vi "solar_visa VISA Open.vi"(6 "Access Mode (0)":T1 items=["VISA Defaults"=0, "Exclusive Lock"=1, "Load Configured Settings"=4], 8 "error in (no error)":errorcluster, 9 "VISA Close? (T)":bool=TRUE, 10 "VISA Timeout (0 = Ignore)":u32, 11 "VISA Resource in":refnum<visa-resource-name>) -> (0 "error out":errorcluster, 3 "VISA Resource out":refnum<visa-resource-name>)   [LabVIEW 2018]
doc: "This opens a VISA session. \nIf <b>VISA Close?</b> is true the previous VISA session is closed. \nIf <b>VISA Timeout</b> is greater than 0 the VISA timeout is set."
uses:
  <vilib>/Instr/_visa.llb/VISA Open Access Mode.ctl
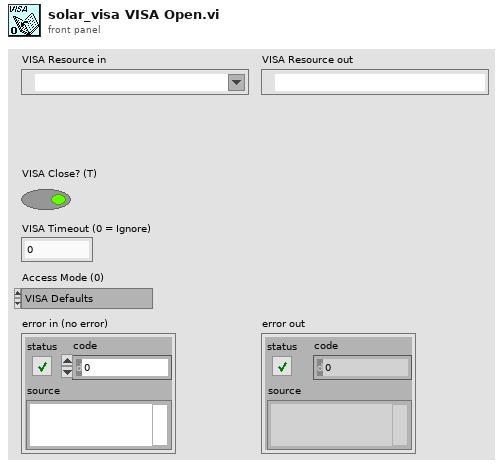
[diagram p1: front panel]
types:
  T1 = typedef "VISA Open Access Mode.ctl" = u32
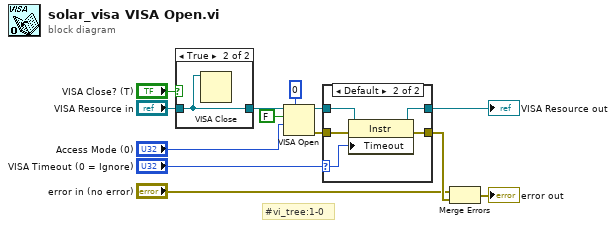
[diagram p0: block diagram]
diagram:
  # "#vi_tree:1-0"
  n1 = case shown="True" "VISA Close? (T)" {
    tunnel: "VISA Resource in" -> [w14 w15]
    tunnel: [w14 w15] -> w2
    frame False {
    }
    frame True {
      n2 = VISA Close(VISA resource name=w15) -> ()  [unwired: 1 in, 1 out]
    }
  }
  n3 = VISA Open(timeout (0)=u32 0 ("VISA Open timeout (0)"), duplicate session (F)=FALSE, access mode="Access Mode (0)", VISA resource name=w2) -> (VISA resource name=w1:refnum<visa-resource-name>, error out=w5:errorcluster)  [unwired: 1 in]
  n4 = case shown="Default" "VISA Timeout (0 = Ignore)" {
    selector: "VISA Timeout (0 = Ignore)" -> [_ w18]
    tunnel: w5 -> [w16 w22]
    tunnel: [w16 w21] -> w10
    tunnel: w1 -> [w17 w20]
    tunnel: [w17 w19] -> w9
    frame 0 {
    }
    frame Default {
      n5 = property class="Instr"(reference=w20, error in=w22, "Timeout"=w18) -> (reference out=w19:refnum<visa-resource-name>, error out=w21:errorcluster)
    }
  }
  "VISA Resource out" <- w9
  n6 = Merge Errors("error in (no error)", w10) -> (→"error out":errorcluster)
